vi "Interpolate Values.vi"(6 "Digital":bool, 8 "Values":dbl[](array[numeric]), 9 "Remaining Time":dbl, 10 "Time in Step":dbl, 11 "Duration":dbl) -> (3 "Value Out":dbl)   [LabVIEW 2020, in "Sequencer with Output Values.lvlib" / "Sequencer with Output Values.lvclass"]
uses:
  Sequencer with Output Values.lvclass
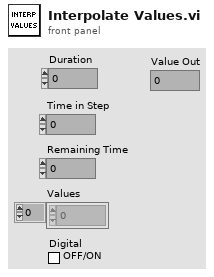
[diagram p1: front panel]
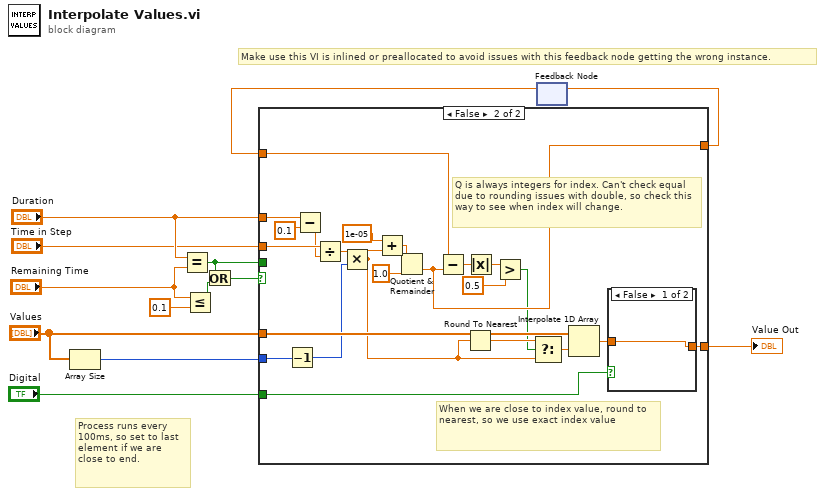
[diagram p0: block diagram]
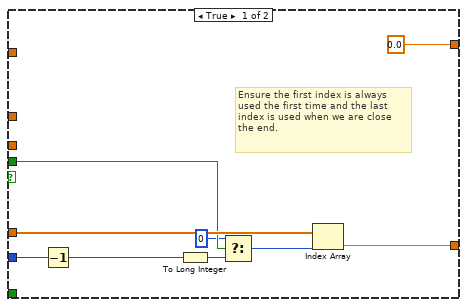
[diagram p2: hidden frame]
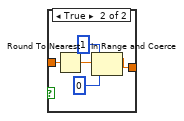
[diagram p3: hidden frame]
diagram:
  # "Make use this VI is inlined or preallocated to avoid issues with this feedback node getting the wrong instance."
  # "Process runs every 100ms, so set to last element if we are close to end."
  n1 = Array Size(array="Values") -> (size(s)=w7:i32)
  n2 = Equal?(x="Duration", y="Remaining Time") -> (x = y?=w6:bool)
  n3 = Less Or Equal?(x="Remaining Time", y=0.1) -> (x <= y?=w3:bool)
  n4 = Or(x=w6, y=w3) -> (x .or. y?=w5:bool)
  n5 = feedback #1() -> (w1:dbl)  [unwired: 1 in]
  n6 = case shown="False" w5 {
    tunnel: "Values" -> [w22 w45]
    tunnel: w7 -> [w16 w43]
    tunnel: "Duration" -> [_ w37]
    tunnel: "Time in Step" -> [_ w41]
    tunnel: [w19 w38] -> w10
    tunnel: w6 -> [w21 _]
    tunnel: "Digital" -> [_ w40]
    tunnel: [0.0 w30] -> w2
    tunnel: w1 -> [_ w31]
    frame True {
      # "Ensure the first index is always used the first time and the last index is used when we are close the end."
      n7 = Decrement(x=w16) -> (x-1=w15:i32)
      n8 = To Long Integer(number=w15) -> (32bit integer=w17:i32)
      n9 = Select(t=0 ("f"), s=w21, f=w17) -> (s? t:f=w20:i32)
      n10 = Index Array(array=w22, index=w20) -> (element=w19:dbl)
    }
    frame False {
      # "Q is always integers for index. Can't check equal due to rounding issues with double, so check this way to see when index will change."
      # "When we are close to index value, round to nearest, so we use exact index value"
      n11 = Decrement(x=w43) -> (x-1=w42:i32)
      n12 = Subtract(x=w37, y=0.1) -> (x-y=w35:dbl)
      n13 = Divide(x=w41, y=w35) -> (x/y=w44:dbl)
      n14 = Multiply(x=w44, y=w42) -> (x*y=w25:dbl)
      n15 = Add(x=1e-05, y=w25) -> (x+y=w23:dbl)
      n16 = Quotient & Remainder(x=w23, y=1.0) -> (floor(x/y)=w30:dbl)  [unwired: 1 out]
      n17 = Subtract(x=w31, y=w30) -> (x-y=w29:dbl)
      n18 = Round To Nearest(number=w25) -> (nearest integer value=w33:dbl)
      n19 = Absolute Value(x=w29) -> (abs(x)=w28:dbl)
      n20 = Greater?(x=w28, y=0.5) -> (0:w26:bool)
      n21 = Select(t=w33, s=w26, f=w25) -> (s? t:f=w32:dbl)
      n22 = Interpolate 1D Array(1:w32, 2:w45) -> (0:w39:dbl)
      n23 = case shown="False" w40 {
        tunnel: w39 -> [w46 w51]
        tunnel: [w46 w49] -> w38
        frame False {
        }
        frame True {
          n24 = Round To Nearest(number=w51) -> (nearest integer value=w50:dbl)
          n25 = In Range and Coerce(upper limit=1, x=w50, lower limit=0) -> (coerced(x)=w49:dbl)  [unwired: 1 out]
        }
      }
    }
  }
  "Value Out" <- w10
  n26 = feedback-in #1(w2) -> ()
